vi "Add.vi"(8 "error in (no error)":errorcluster, 9 "Value":refnum<class>, 10 "Key":string, 11 "Array In":refnum<class "Array.lvclass">) -> (0 "error out":errorcluster, 3 "Array Out":refnum<class "Array.lvclass">)   [LabVIEW 2013, in "LapDog.Collections.v1.Maps.Implementations.lvlib" / "Array.lvclass"]
doc: "Add a key-value pair to the map.\n\nIf the key already exists, error 510202 is returned."
uses:
  Array.lvclass
  Array.lvclass/Array.ctl
  LapDog.Collections.Common/LapDog.Collections.v1.Common.lvlib
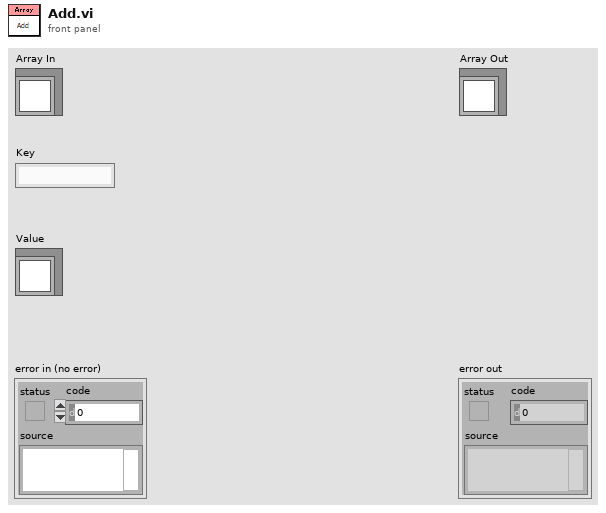
[diagram p1: front panel]
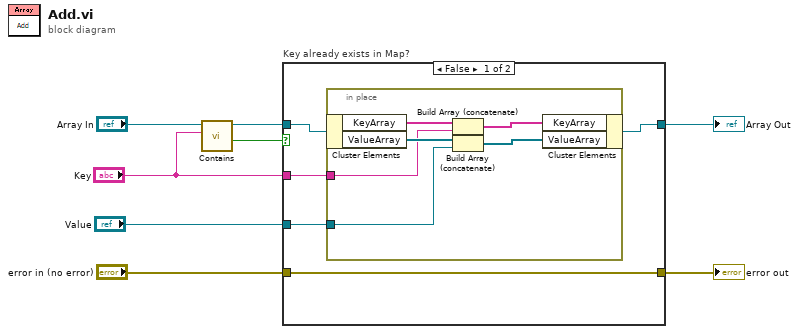
[diagram p0: block diagram]
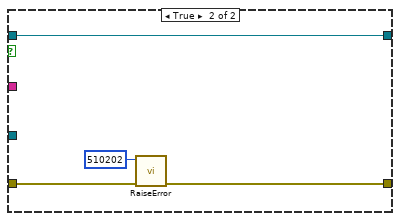
[diagram p2: hidden frame]
diagram:
  n1 = call-dynamic "Contains.vi"("Key"="Key", "Array In"="Array In") -> ("Key Exists?"=w6:bool, "Array Out"=w7:refnum<class "Array.lvclass">)  [unwired: 7 in, 1 out]
  n2 = case "Key already exists in Map?" shown="False" w6 {
    tunnel: [w12 w23] -> w2
    tunnel: w7 -> [w13 w23]
    tunnel: "Value" -> [w11 _]
    tunnel: "error in (no error)" -> [w9 w22]
    tunnel: [w9 w21] -> w3
    tunnel: "Key" -> [w10 _]
    frame False {
      n3 = in-place {
        in-place-border: w11 -> [w14]
        in-place-border: w10 -> [w15]
        n4 = in-place-cluster #1(w13) -> ("KeyArray"=w18:string[], "ValueArray"=w19:refnum<class>[])
        n5 = Build Array (concatenate)(w18, w15) -> (w17:string[])
        n6 = Build Array (concatenate)(w19, w14) -> (w16:refnum<class>[])
        n7 = in-place-cluster #1("KeyArray"=w17, "ValueArray"=w16) -> (w12:refnum<class "Array.lvclass">)
      }
    }
    frame True {
      n8 = call "RaiseError.vi"("error in (no error)"=w22, "Error Code"=510202) -> ("error out"=w21:errorcluster)  [unwired: 9 in]
    }
  }
  "error out" <- w3
  "Array Out" <- w2
